vi "Sandbox.vi"() -> ()   [LabVIEW 2018, in "Sandbox.lvlib"]
uses:
  Sandbox.lvlib
  Loop Control.xctl
  <vilib>/Platform/TimedLoop/XDataNode/timing_clust.ctl
  <vilib>/Platform/TimedLoop/XDataNode/nitl_modes.ctl
  <vilib>/Platform/TimedLoop/XDataNode/wakeup.ctl
  <vilib>/platform/TimedLoop/XDataNode/XDataNode.xnode
  <vilib>/Platform/TimedLoop/XDataNode/XDNodeRunTimeDep.lvlib
panel:
  out "Waveform Chart":dynamicdata(graph)
  in  "Loop Control":T1(xcontrol)
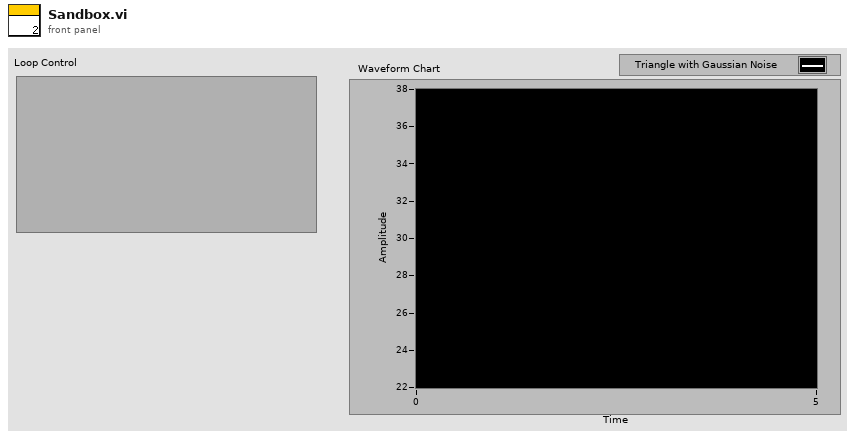
[diagram p1: front panel]
types:
  T1 = cluster{"dt":i64, "error to show":errorcluster, "Active":bool, "stop":bool}
  T2 = typedef "XDNodeRunTimeDep.lvlib/timing_clust.ctl" = cluster{"Expected End [f-1]":u64, "Actual End [f-1]":u64, "Finished Late? [f-1]":bool, "Expected End [i-1]":u64, "Actual End [i-1]":u64, "Finished Late? [i-1]":bool, "Expected Start [i]":u64, "Actual Start [i]":u64, "Expected Start [f]":u64, "Actual Start [f]":u64, "Source Name":string, "Structure Name":string, "Period":i64, "Deadline":i64, "Offset":i64, "Start":i64, "Priority":i32, "Timeout":i32, "Mode":T3, "Wakeup Reason":T4, "Error":errorcluster, "Source Type":string, "Secondary Source Type":string, "Global End Time":u64, "Global Start Time":u64, "Frame Duration":u64, "Iteration Duration":u64, "Assigned CPU":i32, "I/O Scan Engine Mode":u32}
  T3 = typedef "XDNodeRunTimeDep.lvlib/nitl_modes.ctl" = enum32{"No Change", "Process missed periods, maintain original phase", "Discard missed periods, maintain original phase", "Process missed periods, ignore original phase", "Discard missed periods, ignore original phase"}
  T4 = typedef "XDNodeRunTimeDep.lvlib/wakeup.ctl" = enum32{"Normal", "Aborted", "Asynchronous wakeup", "Timing source error", "Timed loop error", "Timeout"}
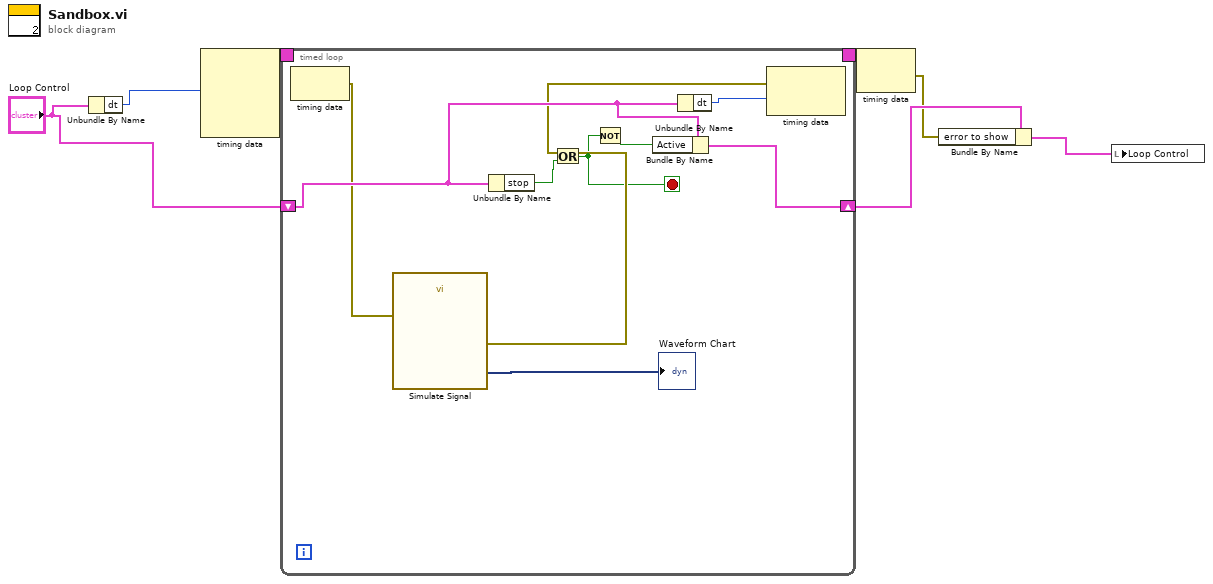
[diagram p0: block diagram]
diagram:
  n1 = Unbundle By Name("Loop Control") -> ("dt"=w5:i64)
  n2 = node-c288(w5) -> (w7:T2)  [unwired: 3 in]
  n3 = timed-loop {
    timing: w7 -> [_]
    timing-out: [_] -> w6
    shift-right: [w12] -> w3
    shift-left: "Loop Control" -> [w13]
    stop <- w9 stop-if-true
    n4 = node-c288() -> (w8:errorcluster)  [unwired: 1 in]
    n5 = call "Simulate Signal"("error in (no error)"=w8) -> ("Triangle with Gaussian Noise"=→"Waveform Chart":dynamicdata, "error out"=w10:errorcluster)  [unwired: 13 in]
    n6 = Unbundle By Name(w13) -> ("stop"=w16:bool)
    n7 = Or(x=w10, y=w16) -> (x .or. y?=w9:bool)
    n8 = Not(x=w9) -> (.not. x?=w15:bool)
    n9 = Bundle By Name(cluster=w13, "Active"=w15) -> (w12:T1)
    n10 = Unbundle By Name(w13) -> ("dt"=w14:i64)
    n11 = node-c288(w10, w14) -> ()  [unwired: 1 out]
  }
  n12 = node-c288(w6) -> (w2:errorcluster)
  n13 = Bundle By Name(cluster=w3, "error to show"=w2) -> (w1:T1)
  n14 = local write "Loop Control"(w1) -> ()
